vi "saving_waveform.vi"(8 "error in (no error)":errorcluster, 9 "Array":waveform(dbl)[](array[waveform]), 10 "directory":path, 11 "Massa":string="_") -> (0 "error out":errorcluster)   [LabVIEW 2017]
uses:
  <vilib>/Waveform/WDTFileIO.llb/Export Waveforms To Spreadsheet File (1D).vi
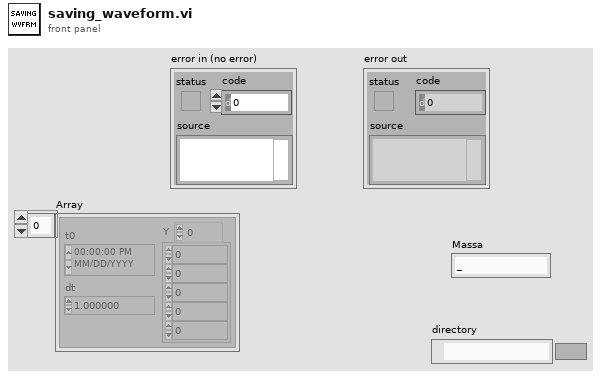
[diagram p1: front panel]
types:
  T1 = enum16{"open", "replace", "create", "open or create", "replace or create", "replace or create with confirmation"}
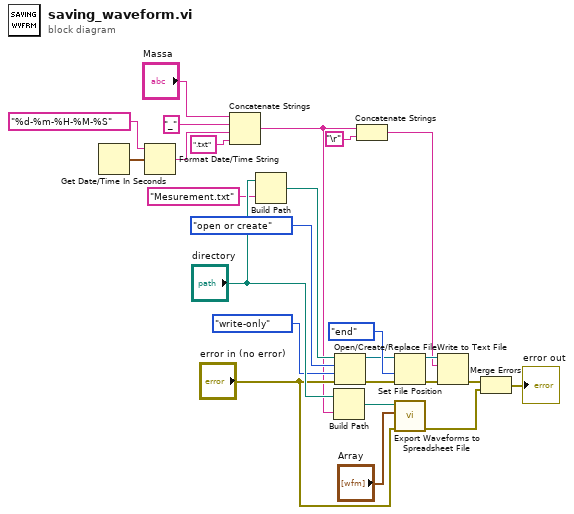
[diagram p0: block diagram]
diagram:
  n1 = Get Date/Time In Seconds() -> (seconds since 1Jan1904=w23:timestamp)
  n2 = Format Date/Time String(time format string (%c)="%d-%m-%H-%M-%S", seconds (now)=w23) -> (date/time string=w25:string)  [unwired: 1 in]
  n3 = Concatenate Strings("Massa", "_" ("Peso 2"), w25, ".txt" ("Peso 2")) -> (w3:string)
  n4 = Build Path(base path="directory", name or relative path="Mesurement.txt") -> (appended path=w15:path)
  n5 = Build Path(base path="directory", name or relative path=w3) -> (appended path=w19:path)
  n6 = Open/Create/Replace File(file path (use dialog)=w15, error in="error in (no error)", operation (0:open)=T1."open or create", access (0:read/write)=enum16{"read/write", "read-only", "write-only"}."write-only") -> (refnum out=w11:refnum<file>, error out=w9:errorcluster)  [unwired: 2 in, 1 out]
  n7 = Concatenate Strings(w3, "\r") -> (w2:string)
  n8 = Set File Position(refnum=w11, from (0:start)=enum16{"start", "end", "current"}."end", error in=w9) -> (refnum out=w13:refnum<file>, error out=w14:errorcluster)  [unwired: 1 in]
  n9 = call-poly <vilib>:"Export Waveforms to Spreadsheet File.vi"("error in (no error)"="error in (no error)", "waveforms"="Array", "file path (dialog if empty)"=w19) -> ("error out"=w7:errorcluster)  [unwired: 7 in, 1 out]
  n10 = Write to Text File(file (use dialog)=w13, text=w2, error in=w14) -> (error out=w8:errorcluster)  [unwired: 1 in, 2 out]
  n11 = Merge Errors(w8, w7) -> (→"error out":errorcluster)
